vi "buildDelimitedItemString.vi"(9 "Child":string, 10 "Parent":string, 11 "Root":string) -> (2 "Delimited Item String":string)   [LabVIEW 2017, in "BuildServer.lvlib" / "BuildServer.lvclass"]
uses:
  BuildServer.lvclass
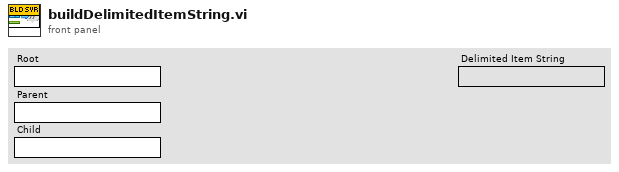
[diagram p1: front panel]
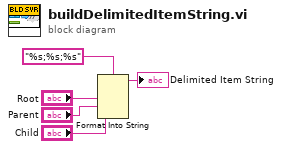
[diagram p0: block diagram]
diagram:
  n1 = Format Into String(format string="%s;%s;%s", "Root", "Parent", "Child") -> (resulting string=→"Delimited Item String":string)  [unwired: 2 in, 1 out]
